vi "Error Query.vi"(8 "error in (no error)":errorcluster, 11 "VISA resource name":refnum<visa-resource-name>) -> (0 "error out":errorcluster, 2 "Error":bool, 3 "VISA resource name out":refnum<visa-resource-name>)   [LabVIEW 2011, in "Ocean Server OS4000.lvlib"]
doc: "Parses the data sent by the instrument to check if there is any error."
uses:
  Ocean Server OS4000.lvlib
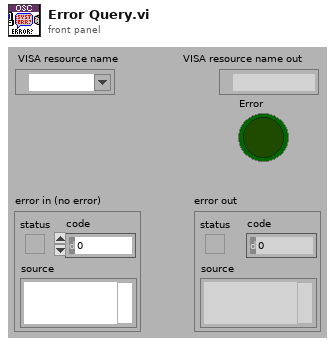
[diagram p1: front panel]
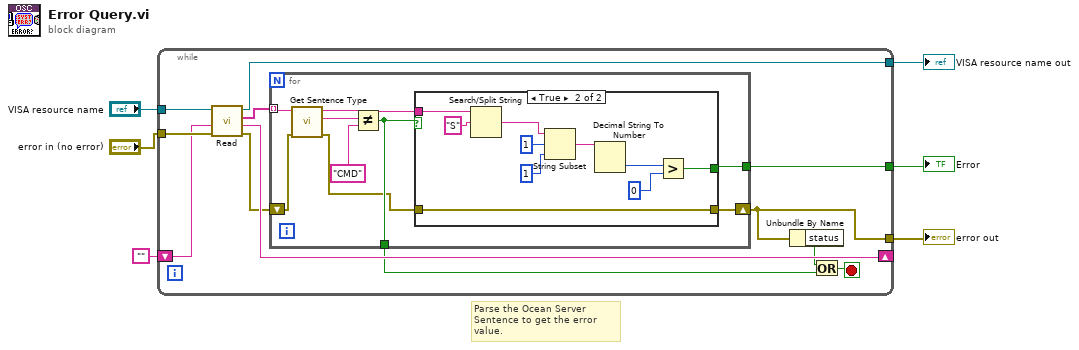
[diagram p0: block diagram]
diagram:
  # "Parse the Ocean Server Sentence to get the error value."
  n1 = while {
    tunnel: "VISA resource name" -> [w18]
    tunnel: "error in (no error)" -> [w17]
    shift-right: [w15] -> _
    shift-left: "" ("Remaining Sentence") -> [w14]
    tunnel: [w7] -> w1
    tunnel: [w12] -> w2
    tunnel: [w9] -> w4
    stop <- w11 stop-if-true
    n2 = call "Read.vi"("error in (no error)"=w17, "Text to prepend to sentence"=w14, "VISA resource name"=w18) -> ("error out"=w13:errorcluster, "Remaining Sentence"=w15:string, "Ocean Server Sentences"=w16:string[], "VISA resource name out"=w12:refnum<visa-resource-name>)  [unwired: 5 in]
    n3 = for {
      tunnel: w16 -> [w27] mode=indexing
      tunnel: [w22] -> w9
      tunnel: [w21] -> w8
      shift-right: [w19] -> w7
      shift-left: w13 -> [w23]
      n4 = call "Get Sentence Type.vi"("error in (no error)"=w23, "Sentence In"=w27) -> ("error out"=w20:errorcluster, "Sentence Type"=w26:string, "Sentence Out"=w24:string)  [unwired: 7 in]
      n5 = Not Equal?(x=w26, y="CMD") -> (x != y?=w21:bool)
      n6 = case shown="True" w21 {
        selector: w21 -> [w29 _]
        tunnel: w24 -> [_ w39]
        tunnel: [w28 w30] -> w19
        tunnel: [w29 w32] -> w22
        tunnel: w20 -> [w28 w30]
        frame False {
        }
        frame True {
          n7 = Search/Split String(string=w39, search string/char (-)="S") -> (match + rest of string=w37:string)  [unwired: 1 in, 2 out]
          n8 = String Subset(string=w37, offset (0)=1, length (rest)=1 ("length (rest)")) -> (substring=w35:string)
          n9 = Decimal String To Number(string=w35) -> (number=w34:i32)  [unwired: 2 in, 1 out]
          n10 = Greater?(x=w34, y=0) -> (0:w32:bool)
        }
      }
    }
    n11 = Unbundle By Name(w7) -> ("status"=w10:bool)
    n12 = Or(x=w10, y=w8) -> (x .or. y?=w11:bool)
  }
  "VISA resource name out" <- w2
  "error out" <- w1
  "Error" <- w4
